vi "Değişkenleri Sıfırla.vi"(8 "error in (no error)":errorcluster) -> (0 "error out":errorcluster)   [LabVIEW 2014]
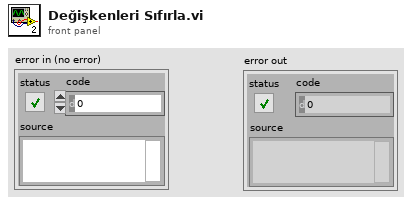
[diagram p1: front panel]
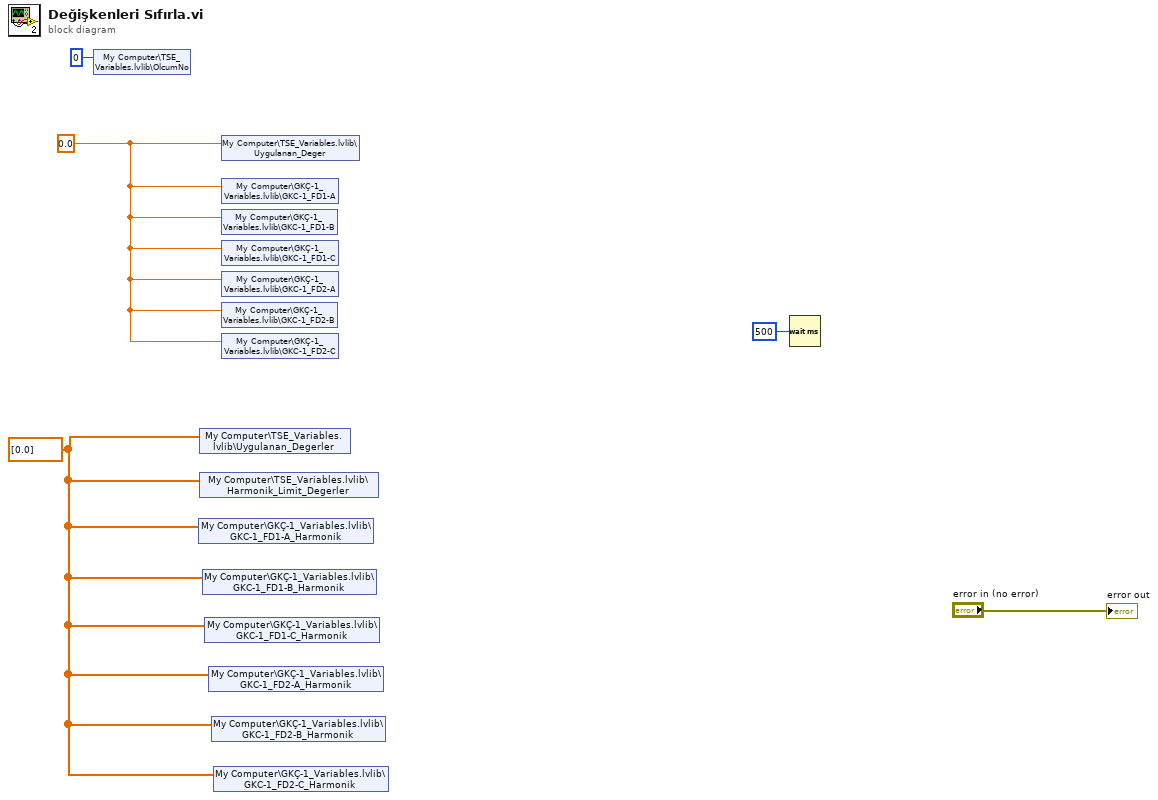
[diagram p0: block diagram]
diagram:
  w3 = 0.0 ("Numeric")
  w1 = dbl[] [0.0] ("Harmonik Limit Değerler")
  n1 = shared-variable "My Computer\\TSE_Variables.lvlib\\OlcumNo"(u16 0 ("OlcumNo")) -> ()  [unwired: 1 in, 1 out]
  n2 = shared-variable "My Computer\\GKÇ-1_Variables.lvlib\\GKC-1_FD1-A_Harmonik"(w1) -> ()  [unwired: 1 in, 1 out]
  n3 = shared-variable "My Computer\\TSE_Variables.lvlib\\Uygulanan_Degerler"(w1) -> ()  [unwired: 1 in, 1 out]
  n4 = shared-variable "My Computer\\TSE_Variables.lvlib\\Harmonik_Limit_Degerler"(w1) -> ()  [unwired: 1 in, 1 out]
  n5 = shared-variable "My Computer\\GKÇ-1_Variables.lvlib\\GKC-1_FD1-B_Harmonik"(w1) -> ()  [unwired: 1 in, 1 out]
  n6 = shared-variable "My Computer\\GKÇ-1_Variables.lvlib\\GKC-1_FD1-C_Harmonik"(w1) -> ()  [unwired: 1 in, 1 out]
  n7 = shared-variable "My Computer\\GKÇ-1_Variables.lvlib\\GKC-1_FD2-A_Harmonik"(w1) -> ()  [unwired: 1 in, 1 out]
  n8 = shared-variable "My Computer\\GKÇ-1_Variables.lvlib\\GKC-1_FD2-B_Harmonik"(w1) -> ()  [unwired: 1 in, 1 out]
  n9 = shared-variable "My Computer\\GKÇ-1_Variables.lvlib\\GKC-1_FD2-C_Harmonik"(w1) -> ()  [unwired: 1 in, 1 out]
  n10 = shared-variable "My Computer\\TSE_Variables.lvlib\\Uygulanan_Deger"(w3) -> ()  [unwired: 1 in, 1 out]
  n11 = shared-variable "My Computer\\GKÇ-1_Variables.lvlib\\GKC-1_FD1-A"(w3) -> ()  [unwired: 1 in, 1 out]
  n12 = shared-variable "My Computer\\GKÇ-1_Variables.lvlib\\GKC-1_FD1-B"(w3) -> ()  [unwired: 1 in, 1 out]
  n13 = shared-variable "My Computer\\GKÇ-1_Variables.lvlib\\GKC-1_FD1-C"(w3) -> ()  [unwired: 1 in, 1 out]
  n14 = shared-variable "My Computer\\GKÇ-1_Variables.lvlib\\GKC-1_FD2-A"(w3) -> ()  [unwired: 1 in, 1 out]
  n15 = shared-variable "My Computer\\GKÇ-1_Variables.lvlib\\GKC-1_FD2-B"(w3) -> ()  [unwired: 1 in, 1 out]
  n16 = shared-variable "My Computer\\GKÇ-1_Variables.lvlib\\GKC-1_FD2-C"(w3) -> ()  [unwired: 1 in, 1 out]
  n17 = Wait (ms)(milliseconds to wait=u32 500) -> ()  [unwired: 1 out]
  "error out" <- "error in (no error)"
